vi "Export to Matlab.vi"(7 "Display?":bool, 8 "error in (no error)":errorcluster, 11 "Log file path":path) -> (0 "error out":errorcluster)   [LabVIEW 2020]
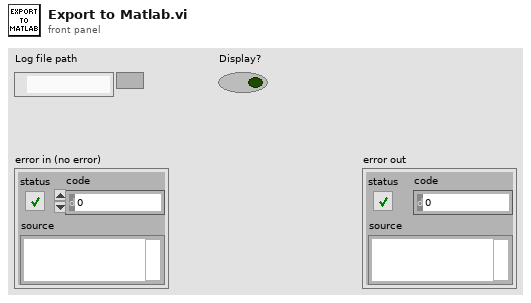
[diagram p1: front panel]
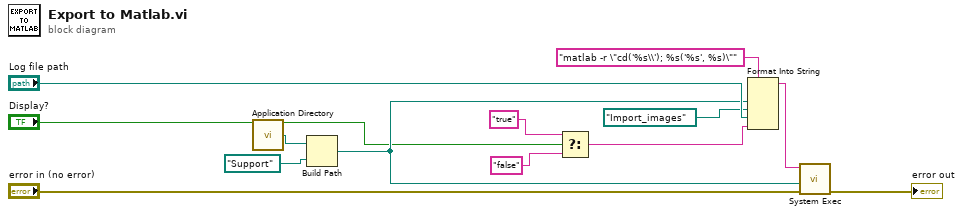
[diagram p0: block diagram]
diagram:
  n1 = call <vilib>:"Application Directory.vi"() -> ("Application Directory"=w4:path)
  n2 = Build Path(base path=w4, name or relative path=path "Support") -> (appended path=w8:path)
  n3 = Select(t="true" ("format string"), s="Display?", f="false" ("format string")) -> (s? t:f=w11:string)
  n4 = Format Into String(format string="matlab -r \"cd('%s\\'); %s('%s', %s)\"", w8, path "Import_images" ("name or relative path"), "Log file path", w11) -> (resulting string=w12:string)  [unwired: 2 in, 1 out]
  n5 = call <vilib>:"System Exec.vi"("error in (no error)"="error in (no error)", "working directory"=w8, "command line"=w12) -> ("error out"=→"error out":errorcluster)  [unwired: 5 in, 3 out]
